vi "Compute DistanceTo AprilTag.vi"(6 "Robot Calibration Cluster":T1={"Camera Height on robot (in)"=34.5, "Camera Angle on the robot (deg)"=28.3, "Camera FOV Top to Bottom View Angle (deg)"=0.946, "Camera FOV Left to Right View Angle (deg)"=26.5, "Target size (in)"=6.5, "Distance to front of bumper (in)"=9.75, "Focal Length (mm)"=10.0} {"Camera FOV Left to Right View Angle (deg)" format="%#_13g"; "Focal Length (mm)" format="%#_13g"; "Distance to front of bumper (in)" format="%#_13g"; "Target size (in)" format="%#_13g"; "Camera FOV Top to Bottom View Angle (deg)" format="%#_13g"; "Camera Angle on the robot (deg)" format="%#_13g"; "Camera Height on robot (in)" format="%#_13g"}, 8 "results":T2={"diameter points"={"first point"={"x"=0.0, "y"=0.0}, "projected point"={"x"=0.0, "y"=0.0}}, "normalized center"={"x"=0.0, "y"=0.0}, "Overall Score"=0.0, "Distance (ft)"=0.0, "Offset Angle"=0.0, "Tag corner points"=[], "Tag Center"={"X"=0.0, "Y"=0.0}, "Tag Yaw"=0.0, "Tag Pitch"=0.0, "Target Roll (deg)"=0.0, "AprilTag Number"=68} {"Tag Center"."Y" format="%0.2f"; "Tag Center"."X" format="%0.2f"}, 11 "Image Src":T3) -> (0 "results out":T2={"diameter points"={"first point"={"x"=0.0, "y"=0.0}, "projected point"={"x"=0.0, "y"=0.0}}, "normalized center"={"x"=0.0, "y"=0.0}, "Overall Score"=0.0, "Distance (ft)"=0.0, "Offset Angle"=0.0, "Tag corner points"=[], "Tag Center"={"X"=0.0, "Y"=0.0}, "Tag Yaw"=0.0, "Tag Pitch"=0.0, "Target Roll (deg)"=0.0, "AprilTag Number"=68} {"Tag Center"."Y" format="%0.2f"; "Tag Center"."X" format="%0.2f"}, 1 "Target Yaw (deg)":dbl, 2 "Offset Angle":dbl=569.258018632146, 3 "Image Dst Out":T3, 4 "Distance from target (in)":dbl=116.40675998176638 format="%.2f", 5 "Target Pitch (deg)":dbl)   [LabVIEW 2023]
doc: "Using the camera lens information and the real world size of the target, use trig and ratios to determine the distance to the target. Also returns the location relative to the image center in a (-1 , 1) coordinate system that may be useful for steering the robot."
uses:
  <vilib>/vision/Image Controls.llb/IMAQ Image.ctl
  AprilTag Target Fields.ctl
  Camera Info.ctl
panel:
  out "Target Roll (deg)":dbl
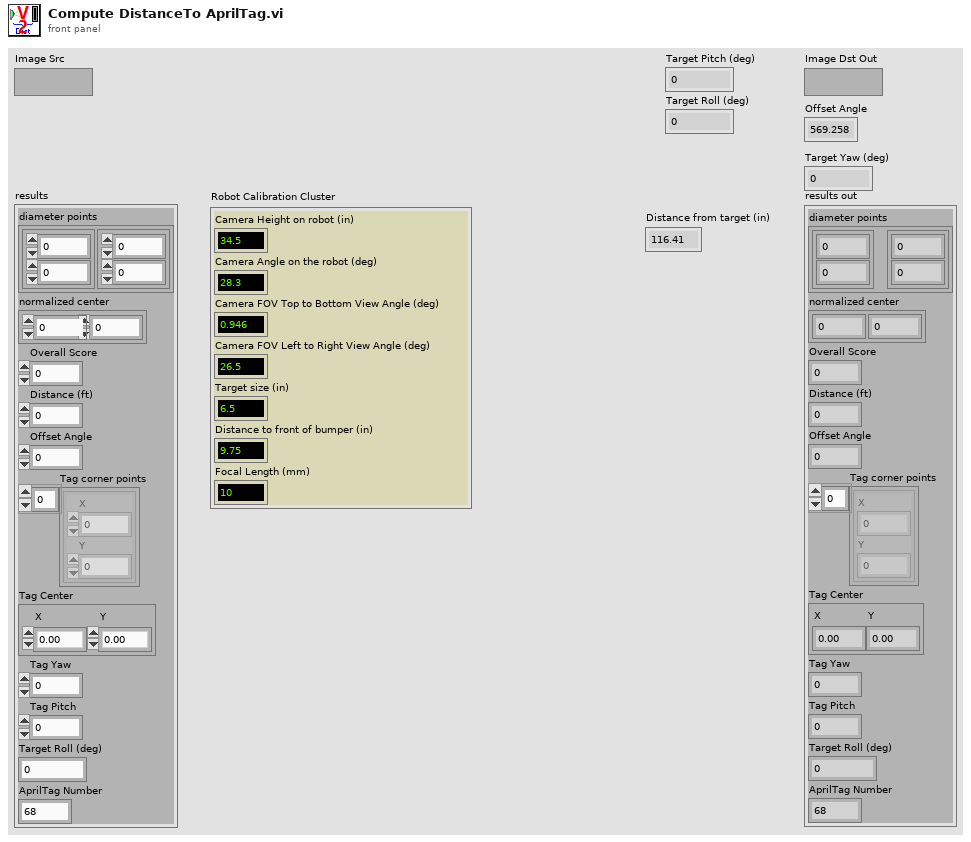
[diagram p1: front panel]
types:
  T1 = typedef "Camera Info.ctl" = cluster{"Camera Height on robot (in)":dbl, "Camera Angle on the robot (deg)":dbl, "Camera FOV Top to Bottom View Angle (deg)":dbl, "Camera FOV Left to Right View Angle (deg)":dbl, "Target size (in)":dbl, "Distance to front of bumper (in)":dbl, "Focal Length (mm)":dbl}
  T2 = typedef "AprilTag Target Fields.ctl" = cluster{"diameter points":cluster{"first point":cluster{"x":dbl, "y":dbl}, "projected point":cluster{"x":dbl, "y":dbl}}, "normalized center":cluster{"x":dbl, "y":dbl}, "Overall Score":dbl, "Distance (ft)":dbl, "Offset Angle":dbl, "Tag corner points":cluster{"X":dbl, "Y":dbl}[], "Tag Center":cluster{"X":dbl, "Y":dbl}, "Tag Yaw":dbl, "Tag Pitch":dbl, "Target Roll (deg)":dbl, "AprilTag Number":i32}
  T3 = typedef "IMAQ Image.ctl" = refnum<image>
  T4 = cluster{"first point":cluster{"x":dbl, "y":dbl}, "projected point":cluster{"x":dbl, "y":dbl}}
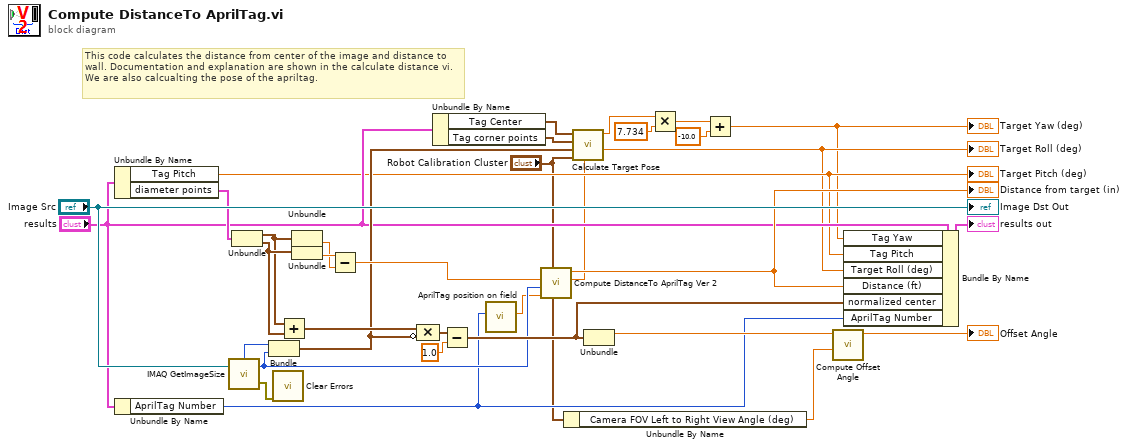
[diagram p0: block diagram]
diagram:
  # "This code calculates the distance from center of the image and distance to wall. Documentation and explanation are shown in the calculate distance vi. We are also calcualting the pose of the apriltag."
  n1 = Unbundle By Name("results") -> ("Tag Pitch"=w10:dbl, "diameter points"=w17:T4)
  "Target Pitch (deg)" <- w10
  n2 = Unbundle By Name("results") -> ("AprilTag Number"=w11:i32)
  n3 = call "IMAQ GetImageSize"("Image"="Image Src") -> ("Y Resolution"=w24:i32, "X Resolution"=w25:i32, "error out"=w34:errorcluster)  [unwired: 3 in]
  n4 = Unbundle(w17) -> ("first point"=w18:cluster{"x":dbl, "y":dbl}, "projected point"=w23:cluster{"x":dbl, "y":dbl})
  n5 = Bundle("X Resolution"=w25, "Y Resolution"=w24) -> (w16:cluster{"X Resolution":i32, "Y Resolution":i32})  [unwired: 1 in]
  n6 = call <vilib>:"Clear Errors.vi"("error in (no error)"=w34) -> ()  [unwired: 5 in, 2 out]
  n7 = Add(x=w18, y=w23) -> (x+y=w30:cluster{"x":dbl, "y":dbl})
  n8 = Unbundle(w18) -> ("y"=w20:dbl)  [unwired: 1 out]
  n9 = Unbundle(w23) -> ("y"=w21:dbl)  [unwired: 1 out]
  n10 = Subtract(x=w21, y=w20) -> (x-y=w19:dbl)
  n11 = Compound Arithmetic op=MULTIPLY(w30, invert w16) -> (w31:cluster{dbl, dbl})
  n12 = Unbundle By Name("results") -> ("Tag Center"=w14:cluster{"X":dbl, "Y":dbl}, "Tag corner points"=w15:cluster{"X":dbl, "Y":dbl}[])
  n13 = Subtract(x=w31, y=1.0) -> (x-y=w28:cluster{dbl, dbl})
  n14 = call "AprilTag position on field.vi"("AprilTag Number"=w11) -> ("Target height to center (in)"=w22:dbl)  [unwired: 10 in]
  n15 = call "Compute DistanceTo AprilTag Ver 2.vi"("Robot Calibration Cluster"="Robot Calibration Cluster", "Height to center of target from floor (hp (in))"=w22, "Screen resolution pixels Height (Ry)"=w24, "Target Vertical pixels bottom - top (pixels)"=w19) -> ("Distance from target to camera (in) 2"=w5:dbl, "Distance from target to bumper (in)"=w13:dbl)  [unwired: 6 in]
  "Distance from target (in)" <- w13
  n16 = Unbundle By Name("Robot Calibration Cluster") -> ("Camera FOV Left to Right View Angle (deg)"=w7:dbl)
  n17 = call "Calculate Target Pose.vi"("Distance to target (in)"=w5, "Robot Calibration Cluster"="Robot Calibration Cluster", "Camera Resolution"=w16, "Corners"=w15, "Target Center"=w14) -> ("Target Roll (deg)"=w9:dbl, "Target Yaw (deg)"=w3:dbl)  [unwired: 4 in, 1 out]
  "Target Roll (deg)" <- w9
  n18 = Unbundle(w28) -> (w27:dbl)  [unwired: 1 out]
  n19 = Multiply(x=w3, y=7.734) -> (x*y=w4:dbl)
  n20 = Add(x=w4, y=-10.0) -> (x+y=w2:dbl)
  "Target Yaw (deg)" <- w2
  n21 = call "Compute Offset Angle.vi"("Field of view"=w7, "Offset Normilized"=w27) -> ("Offset Angle"=→"Offset Angle":dbl)  [unwired: 9 in]
  n22 = Bundle By Name(cluster="results", "Tag Yaw"=w2, "Tag Pitch"=w10, "Target Roll (deg)"=w9, "Distance (ft)"=w13, "normalized center"=w28, "AprilTag Number"=w11) -> (→"results out":T2)
  "Image Dst Out" <- "Image Src"
